vi "OSICS_Module_Identification.vi"(7 "OSICS slot":i32=1 min=1 max=8 step=1, 8 "error in":errorcluster, 11 "VISA IN":refnum<visa-resource-name>) -> (0 "error out":errorcluster, 2 "Module indentification":string, 3 "VISA OUT":refnum<visa-resource-name>, 5 "ERR":i32)   [LabVIEW 2014, in "OSICS_LIB.lvlib"]
doc: "This Vi requests information about OSICS modules. Company name, module name, serial number, software version number (FPGA version)."
uses:
  OSICS_LIB.lvlib
panel:
  # "Basic Function to identify a module in the OSICS"
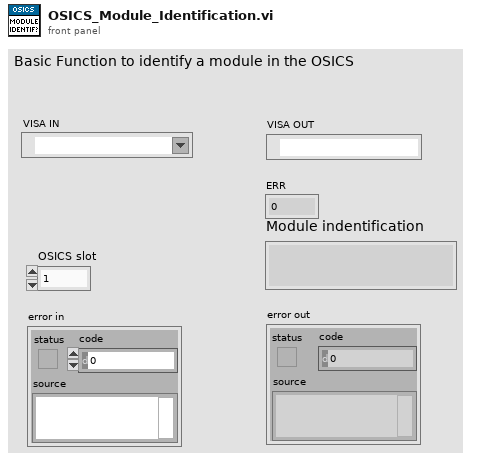
[diagram p1: front panel]
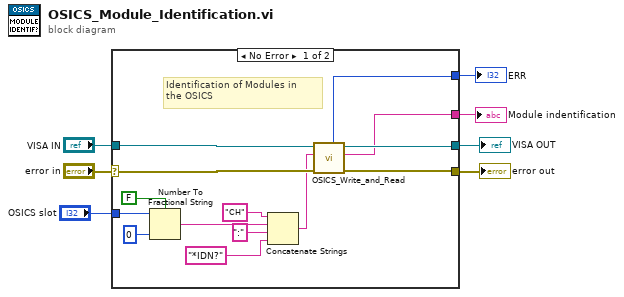
[diagram p0: block diagram]
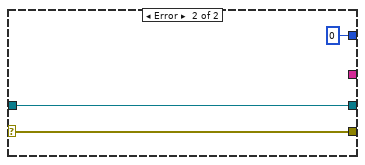
[diagram p2: hidden frame]
diagram:
  n1 = case shown="No Error" "error in" {
    selector: "error in" -> [w20 w23]
    tunnel: "VISA IN" -> [w21 w24]
    tunnel: [w11 w24] -> w6
    tunnel: [w12 w23] -> w5
    tunnel: [w10 0 ("ERR")] -> w3
    tunnel: "OSICS slot" -> [w19 _]
    tunnel: [w8 _] -> w1
    frame No Error {
      # "Identification of Modules in\nthe OSICS"
      n2 = Number To Fractional String(use system decimal point (T)=FALSE, number=w19, precision (6)=i16 0) -> (F-format string=w15:string)  [unwired: 1 in]
      n3 = Concatenate Strings("CH" ("string"), w15, ":" ("string"), "*IDN?" ("string")) -> (w13:string)
      n4 = call "OSICS_Write_and_Read.vi"("error in (no error)"=w20, "String to Send"=w13, "VISA IN"=w21) -> ("error out"=w12:errorcluster, "Message Available"=w8:string, "VISA OUT"=w11:refnum<visa-resource-name>, "ERR"=w10:i32)  [unwired: 5 in]
    }
    frame Error {
    }
  }
  "error out" <- w5
  "VISA OUT" <- w6
  "ERR" <- w3
  "Module indentification" <- w1
